vi "get waveform - 8bit.vi"(8 "error in (no error)":errorcluster caption="에러 입력(에러 없음)", 11 "WAV File 입력":refnum<class "WAV File.lvclass">) -> (0 "error out":errorcluster caption="에러 출력", 1 "8bit memory data":u8[](array[numeric]), 2 "8bit waveform":waveform(i8), 3 "WAV File 출력":refnum<class "WAV File.lvclass">)   [LabVIEW 2020, in "WAV File.lvclass"]
uses:
  WAV File.lvclass
  WAV File.lvclass/WAV File.ctl
  Accessors/Read sound format.vi
  Waveform Obj/Accessors/Read sampling rate.vi
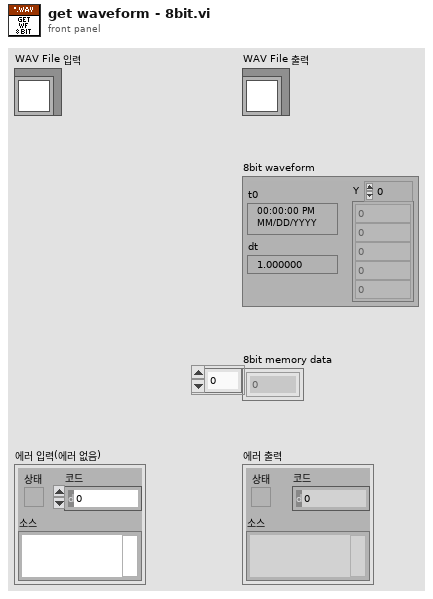
[diagram p1: front panel]
types:
  T1 = typedef "Sound Data Format.ctl" = cluster{"sample rate (S/s)":dbl, "number of channels":i32, "bits per sample":i32}
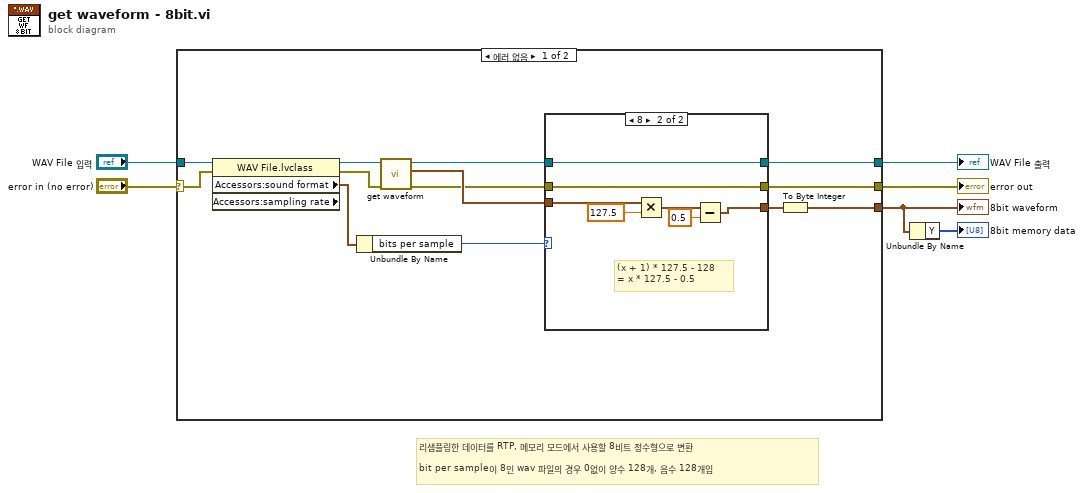
[diagram p0: block diagram]
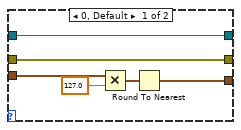
[diagram p2: hidden frame]
diagram:
  # "리샘플링한 데이터를 RTP, 메모리 모드에서 사용할 8비트 정수형으로 변환\n\nbit per sample이 8인 wav 파일의 경우 0없이 양수 128개, 음수 128개임"
  n1 = case shown="에러 없음" "error in (no error)" {
    selector: "error in (no error)" -> [w17 w33]
    tunnel: [w18 w34] -> w5
    tunnel: "WAV File 입력" -> [w13 w34]
    tunnel: [w19 w33] -> w3
    tunnel: [w15 _] -> w2
    frame No Error {
      n2 = property class="WAV File.lvclass" props=["Accessors:sound format", "Accessors:sampling rate"](reference=w13, error in=w17) -> (reference out=w11:refnum<class "WAV File.lvclass">, error out=w14:errorcluster, "Accessors:sound format"=w12:T1)  [unwired: 1 out]
      n3 = Unbundle By Name(w12) -> ("bits per sample"=w9:i32)
      n4 = call-dynamic "get waveform.vi"("error in (no error)"=w14, "WAV File 입력"=w11) -> ("error out"=w7:errorcluster, "waveform"=w8:waveform(dbl), "WAV File 출력"=w10:refnum<class "WAV File.lvclass">)  [unwired: 7 in]
      n5 = case shown="8" w9 {
        tunnel: [w21 w31] -> w19
        tunnel: [w22 w32] -> w18
        tunnel: w10 -> [w22 w32]
        tunnel: w7 -> [w21 w31]
        tunnel: [w23 w26] -> w16
        tunnel: w8 -> [w20 w29]
        frame 0, Default {
          n6 = Multiply(x=w20, y=127.0) -> (x*y=w24:waveform(dbl))
          n7 = Round To Nearest(number=w24) -> (nearest integer value=w23:waveform(dbl))
        }
        frame 8 {
          # "(x + 1) * 127.5 - 128\n= x * 127.5 - 0.5"
          n8 = Multiply(x=w29, y=127.5) -> (x*y=w28:waveform(dbl))
          n9 = Subtract(x=w28, y=0.5) -> (x-y=w26:waveform(dbl))
        }
      }
      n10 = To Byte Integer(number=w16) -> (8bit integer=w15:waveform(i8))
    }
    frame Error {
    }
  }
  "error out" <- w3
  "WAV File 출력" <- w5
  "8bit waveform" <- w2
  n11 = Unbundle By Name(w2) -> ("Y"=→"8bit memory data":i8[])
